vi "DSP48 Counter.vi"(2 "Reset ?":bool, 7 "Increment":bool, 9 "Input Valid":bool=TRUE) -> (8 "Counter Value":fxp<+/-,48,48>, 10 "Output Valid":bool)   [LabVIEW 2012]
doc: "This VI implements 48-bit counter.\n\n<b> Reset : </b> When Reset is done, the counter value becomes zero in the next cycle.\n\nCounter Value gets incremented when increment signal is high.\n\n<b> Latency = 1 Tick </b>\n<b> Resource Usage = 1 DSP48 </b>"
uses:
  <vilib>/rvi/FXPMathLib/basic elements/DSP48E/simVIs/niFpgaDsp48eSimulationState.ctl
  <vilib>/rvi/FXPMathLib/basic elements/DSP48E/subVIs/niFpgaDsp48eType.ctl
  <vilib>/rvi/FXPMathLib/basic elements/DSP48E/subVIs/niFpgaDsp48eAlumodeOpmodeCarryinselState.ctl
  <vilib>/rvi/FXPMathLib/basic elements/DSP48E/subVIs/niFpgaDsp48eUseMultiplierState.ctl
  <vilib>/rvi/FXPMathLib/basic elements/DSP48E/subVIs/niFpgaDsp48eLogicUnitModeState.ctl
  <vilib>/rvi/FXPMathLib/basic elements/DSP48E/subVIs/niFpgaDsp48eSelectPatternState.ctl
  <vilib>/rvi/FXPMathLib/basic elements/DSP48E/subVIs/niFpgaDsp48eSelectMaskState.ctl
  <vilib>/rvi/FXPMathLib/basic elements/DSP48E/subVIs/niFpgaDsp48eAutoresetState.ctl
  <vilib>/rvi/FXPMathLib/basic elements/DSP48E/simVIs/niFpgaDsp48eEnables.ctl
  <vilib>/rvi/FXPMathLib/basic elements/DSP48E/simVIs/niFpgaDsp48eRegisters.ctl
  <vilib>/rvi/FXPMathLib/basic elements/DSP48E/simVIs/niFpgaDsp48eSimMultiplier.vi
  <vilib>/rvi/FXPMathLib/basic elements/DSP48E/simVIs/niFpgaDsp48eSimBundleResets.vi
  <vilib>/rvi/FXPMathLib/basic elements/DSP48E/simVIs/niFpgaDsp48eSimArithmetic.vi
  <vilib>/rvi/FXPMathLib/basic elements/DSP48E/simVIs/niFpgaDsp48eSimPatternDetect.vi
  <vilib>/rvi/FXPMathLib/basic elements/DSP48E/simVIs/niFpgaDsp48eSimP.vi
  <vilib>/rvi/FXPMathLib/basic elements/DSP48E/simVIs/niFpgaDsp48eSimUpdateState.vi
  <vilib>/rvi/FXPMathLib/basic elements/DSP48E/simVIs/niFpgaDsp48eCheckMode.vi
  <vilib>/rvi/FXPMathLib/basic elements/DSP48E/simVIs/niFpgaDsp48eReportInvalidMode.vi
  <vilib>/rvi/FXPMathLib/basic elements/FxpDiscreteDelay/XNode/nifxpmath_DiscreteDelay.xnode
  <vilib>/rvi/FXPMathLib/basic elements/DSP48E/XNode/niFpgaDsp48e.xnode
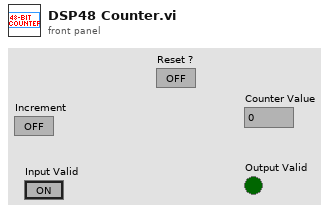
[diagram p1: front panel]
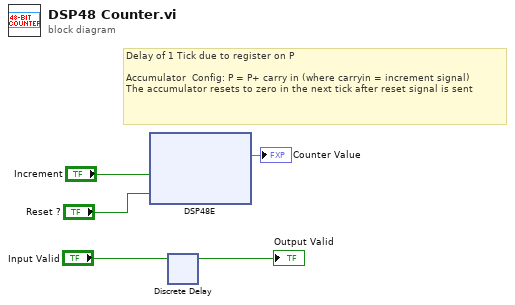
[diagram p0: block diagram]
diagram:
  # "Delay of 1 Tick due to register on P\n\nAccumulator  Config: P = P+ carry in (where carryin = increment signal)\nThe accumulator resets to zero in the next tick after reset signal is sent"
  n1 = xnode "DSP48E"("carryin"="Increment", "clear"="Reset ?") -> ("p"=→"Counter Value":fxp<+/-,48,48>)
  n2 = xnode "Discrete Delay"("D"="Input Valid") -> ("Q"=→"Output Valid":bool)
